vi "Robot Main.vi"() -> ()   [LabVIEW 2016]
doc: "This VI implements the framework and scheduler for your robotics program. It should not be necessary to modify the framework. You are expected to add your code to the VIs called from Robot Main - the ones located in the Team Code folder within the project."
uses:
  <vilib>/Rock Robotics/WPI/Camera/WPI_CameraImageSize.ctl
  <vilib>/Rock Robotics/WPI/ThirdParty/Sensors/navX/_TypeDefs/FRIC_navX_DeviceNumbersTypeDef.ctl
  <vilib>/Rock Robotics/WPI/ThirdParty/Sensors/navX/_Processing Loop/FRIC_navX_Internal_SPI_ProcessingLoop.vi
  Robot Global Data.vi
panel:
  in  "Image Size":T1=enum."320x240"
  in  "Enable Vision":bool
  in  "Finish":bool
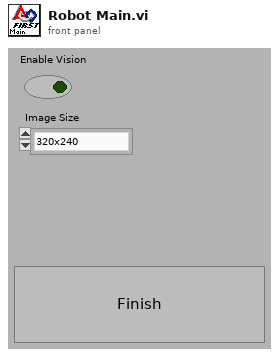
[diagram p1: front panel]
types:
  T1 = typedef "WPI_CameraImageSize.ctl" = enum16{"640x480", "320x240", "160x120", "Custom"}
  T2 = typedef "FRIC_navX_DeviceNumbersTypeDef.ctl" = enum16{"Dev0", "Dev1", "Dev2", "Dev3"}
  T3 = typedef "WPI_DriverStationMatch Info.ctl" = cluster{"Autonomous Elapsed Seconds":dbl, "TeleOp Elapsed Seconds":dbl, "Disabled Elapsed Seconds":dbl, "Visited Autonomous":bool, "Visited TeleOp":bool, "Visited Disabled":bool, "Autonomous Settings":cluster{"Autonomous Style":enum16{"Iterative", "Independent"}, "VI Refnum":refnum<vi>}}
  T4 = typedef "WPI_DriverStationDerivedRobotMode.ctl" = enum16{"Init", "Execute", "Stop"}
  T5 = typedef "WPI_DriverStationRobotMode2.ctl" = enum16{"Autonomous Disabled", "Autonomous Enabled", "Teleop Disabled", "Teleop Enabled", "Disconnected", "Finish", "Test Disabled", "Test Enabled", "Emergency Stopped"}
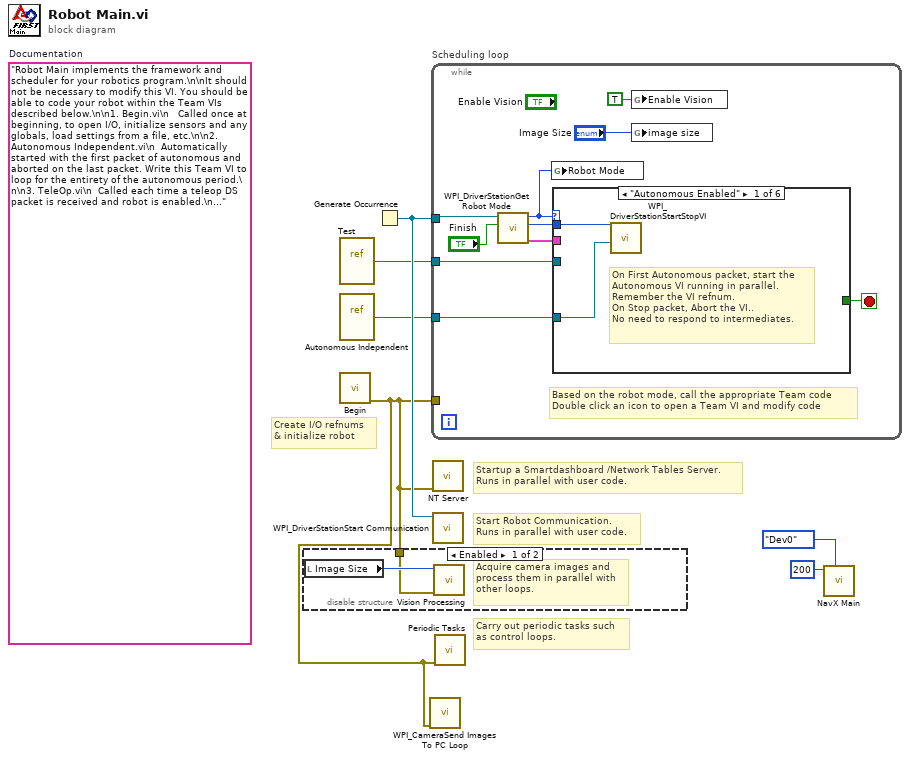
[diagram p0: block diagram]
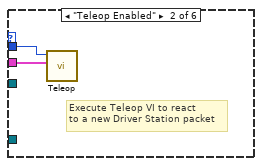
[diagram p3: hidden frame]
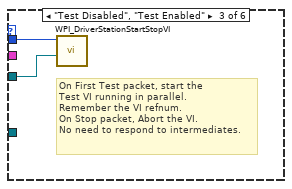
[diagram p4: hidden frame]
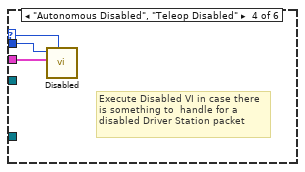
[diagram p5: hidden frame]
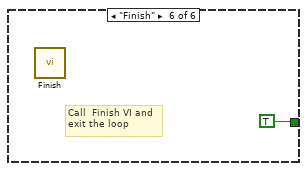
[diagram p7: hidden frame]
diagram:
  (unwired) "Robot Main implements the framework and scheduler for your robotics program.\n\nIt should not be necessary to modify this VI. You should be able to code your robot within the Team VIs described below.\n\n1. Begin.vi\n   Called once at beginning, to open I/O, initialize sensors and any globals, load settings from a file, etc.\n\n2. Autonomous Independent.vi\n  Automatically started with the first packet of autonomous and aborted on the last packet. Write this Team VI to loop for the entirety of the autonomous period.\n\n3. TeleOp.vi\n  Called each time a teleop DS packet is received and robot is enabled.\n\n4. Disabled.vi\n  Called each time a packet is received and the robot is disabled.\n\n5. Test.vi\n  Called Automatically started with the first test packet and aborted on the last. Modify this VI to carry out robot and sensor validation tests.\n\n6. Vision.vi\n  A parallel loop that acquires and processes camera images.\n\n7. PeriodicTasks.vi\n  Parallel loops running at user-defined rates.\n\n8. Finish.vi\n  Called before exiting, so you can save data, clean up I/O, etc.\n"  # Documentation
  # "Startup a Smartdashboard /Network Tables Server.\nRuns in parallel with user code."
  # "Carry out periodic tasks such\nas control loops."
  # "Create I/O refnums\n& initialize robot"
  # "Start Robot Communication.\nRuns in parallel with user code."
  n1 = vi-ref "Test.vi"() -> (w4:refnum<vi>)
  n2 = vi-ref "Autonomous Independent.vi"() -> (w5:refnum<vi>)
  n3 = call "Begin.vi"() -> ("error out"=w1:errorcluster)  [unwired: 2 in, 9 out]
  n4 = disable-structure shown="Enabled" {
    disable-tunnel: w1 -> [w7 _]
    frame Enabled {
      # "Acquire camera images and\nprocess them in parallel with\nother loops."
      n5 = local read "Image Size"() -> (w8:T1)
      n6 = call "Vision Processing.vi"("error in (no error)"=w7, "Image Size"=w8) -> ()  [unwired: 6 out]
    }
    frame Disabled {
    }
  }
  n7 = Generate Occurrence() -> (w6:refnum<k4>)
  n8 = call <vilib>:"WPI_CameraSend Images To PC Loop.vi"("error in (no error)"=w1) -> ()  [unwired: 11 in]
  n9 = while "Scheduling loop" {
    tunnel: w6 -> [w17]
    tunnel: w1 -> [_]
    tunnel: w5 -> [w13]
    tunnel: w4 -> [w11]
    stop <- w14 stop-if-true
    # "Based on the robot mode, call the appropriate Team code\nDouble click an icon to open a Team VI and modify code"
    n10 = call <vilib>:"WPI_DriverStationGet Robot Mode.vi"("Finish"="Finish", "DS Occurrence"=w17) -> ("Match Info out"=w15:T3, "Call Context"=w18:T4, "Robot Mode"=w10:T5)  [unwired: 7 out]
    n11 = global write "Robot Global Data.vi" "Robot Mode"(w10) -> ()
    n12 = case shown="\"Autonomous Enabled\"" w10 {
      selector: w10 -> [_ _ _ w25 _ _]
      tunnel: w18 -> [w20 w22 w24 w27 _ _]
      tunnel: w15 -> [_ w21 _ w26 _ _]
      tunnel: [_ _ _ _ _ TRUE] -> w14
      tunnel: w13 -> [w19 _ _ _ _ _]
      tunnel: w11 -> [_ _ w23 _ _ _]
      frame "Autonomous Enabled" {
        # "On First Autonomous packet, start the\nAutonomous VI running in parallel.\nRemember the VI refnum.\nOn Stop packet, Abort the VI..\nNo need to respond to intermediates."
        n13 = call <vilib>:"WPI_DriverStationStartStopVI.vi"("VI in"=w19, "Call Context"=w20) -> ()  [unwired: 10 in]
      }
      frame "Teleop Enabled" {
        # "Execute Teleop VI to react\nto a new Driver Station packet"
        n14 = call "Teleop.vi"("Match Info"=w21, "Call Context"=w22) -> ()  [unwired: 1 in, 9 out]
      }
      frame "Test Disabled", "Test Enabled" {
        # "On First Test packet, start the\nTest VI running in parallel.\nRemember the VI refnum.\nOn Stop packet, Abort the VI.\nNo need to respond to intermediates."
        n15 = call <vilib>:"WPI_DriverStationStartStopVI.vi"("VI in"=w23, "Call Context"=w24) -> ()  [unwired: 10 in]
      }
      frame "Autonomous Disabled", "Teleop Disabled" {
        # "Execute Disabled VI in case there\nis something to  handle for a\ndisabled Driver Station packet"
        n16 = call "Disabled.vi"("Robot Mode"=w25, "Match Info"=w26, "Call Context"=w27) -> ()  [unwired: 1 in, 8 out]
      }
      frame "Disconnected", Default {
        # "Driver Station packet didn't arrive.\nPossibly useful for diagnostics"
      }
      frame "Finish" {
        # "Call  Finish VI and\nexit the loop"
        n17 = call "Finish.vi"() -> ()  [unwired: 1 in, 7 out]
      }
    }
    n18 = global write "Robot Global Data.vi" "Enable Vision"(TRUE ("Enable Vision")) -> ()
    n19 = global write "Robot Global Data.vi" "image size"("Image Size") -> ()
  }
  n20 = call <vilib>:"NT Server.vi"("error in (no error)"=w1) -> ()  [unwired: 11 in]
  n21 = call <vilib>:"WPI_DriverStationStart Communication.vi"("occurrence"=w6) -> ()  [unwired: 1 in, 10 out]
  n22 = call "Periodic Tasks.vi"("error in"=w1) -> ()  [unwired: 1 in, 10 out]
  n23 = call-poly <vilib>:"NavX Main.vi"("Device Number"=FRIC_navX_DeviceNumbersTypeDef."Dev0", "Rate (4Hz-200Hz)"=u8 200) -> ()  [unwired: 10 in]
